vi "array swap.vi"(10 "search value":string="FEXT", 11 "array":string[](array[string])) -> (3 "swapped array":string[](array[string]))   [LabVIEW 2011]
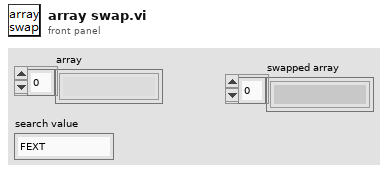
[diagram p1: front panel]
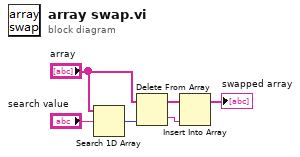
[diagram p0: block diagram]
diagram:
  n1 = Search 1D Array(1D array="array", element="search value") -> (index of element=w6:i32)  [unwired: 1 in]
  n2 = Delete From Array(array="array", index=w6) -> (deleted portion=w4:string, array with subset deleted=w5:string[])  [unwired: 1 in]
  n3 = Insert Into Array(array=w5, new element=w4) -> (→"swapped array":string[])  [unwired: 1 in]
